vi "loadM300MachineStatusYY.vi"(10 "name or relative path":string="M420_LSTR機台狀況(早)_12月.xls", 11 "template (empty)":path=path "c:/m300") -> ()   [LabVIEW 2012]
uses:
  <vilib>/addons/database/Auxilliary.llb/DB Tools Cursor Type.ctl
  <vilib>/Utility/NIReport.llb/NI_report.lvclass
  <vilib>/addons/database/Connection.llb/DB Tools Open Connec (Path).vi
  <vilib>/addons/database/Connection.llb/Conn Execute.vi
  <vilib>/addons/database/Recordset.llb/Rec Destroy - Connection.vi
  <vilib>/addons/_office/excel.llb/Excel Get Data (str).vi
  <vilib>/addons/database/NI_Database_API.lvlib
  <vilib>/addons/_office/NI_ReportGenerationToolkit.lvlib
  <vilib>/Utility/NIReport.llb/Excel/NI_Excel.lvclass
panel:
  out "output cluster":T1
  out "error out 5":errorcluster
  out "error out":errorcluster
  out "after substring":string
  in  "array 2":string[][](array[string])
  in  "Cluster 2":T1
  out "error out 4":errorcluster
  out "error out 3":errorcluster
  in  "start (0, 0)":cluster{"start row":i32, "start column":i32}
  out "x+y":i32
  out "data":string
  in  "start (0, 0) 2":cluster{"start row":i32, "start column":i32}
  out "data 2":string
  in  "start (0, 0) 3":cluster{"start row":i32, "start column":i32}
  out "data 3":string
  out "Numeric":i32
  out "array":string[](array[string])
  out "x+y 2":i32
  out "x > y?":bool
  out "s? t:f":string
  out "concatenated string":string
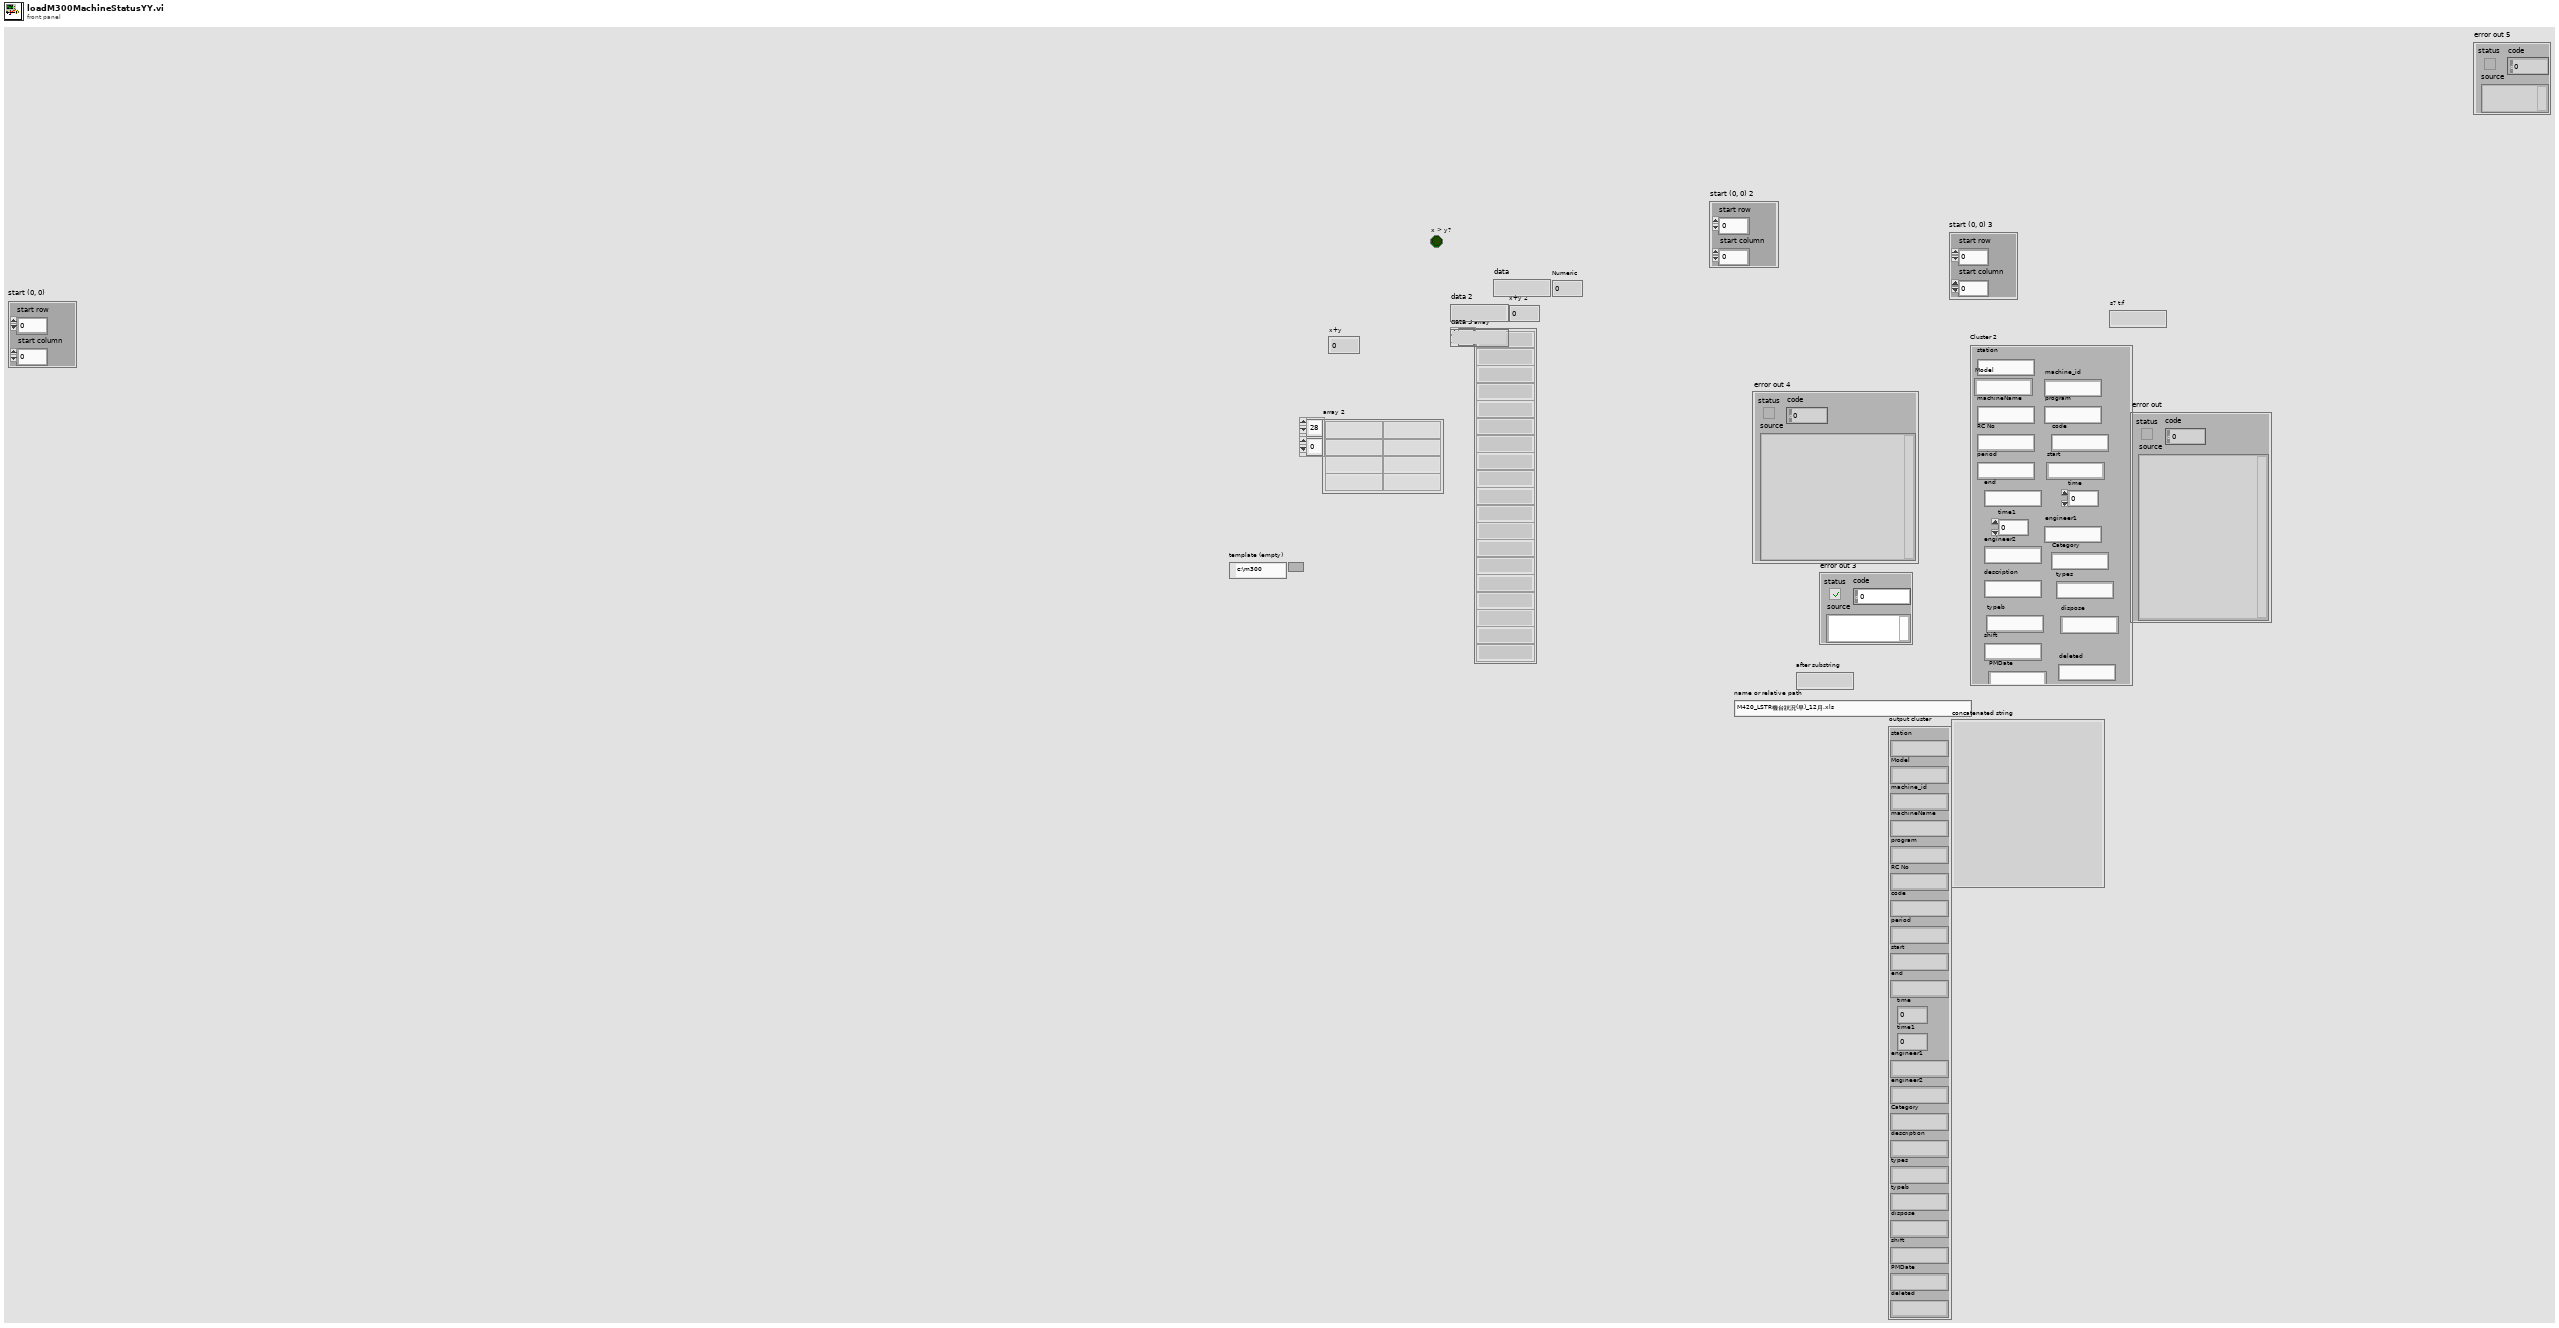
[diagram p1: front panel]
types:
  T1 = cluster{"station":string, "Model":string, "machine_id":string, "machineName":string, "program":string, "RC No":string, "code":string, "period":string, "start":string, "end":string, "time":dbl, "time1":dbl, "engineer1":string, "engineer2":string, "Category":string, "description":string, "types":string, "typeb":string, "dispose":string, "shift":string, "PMDate":string, "deleted":string}
  T2 = enum16{"Standard Report", "HTML", "Word", "Excel"}
  T3 = typedef "NI_Database_API.lvlib/Conn ObjectReference.ctl" = refnum<k1>
  T4 = typedef "NI_Database_API.lvlib/DB Tools Cursor Type.ctl" = enum16{"forward-only", "keyset", "dynamic", "static"}
  T5 = typedef "NI_Database_API.lvlib/Rec ObjectReference.ctl" = refnum<k1>
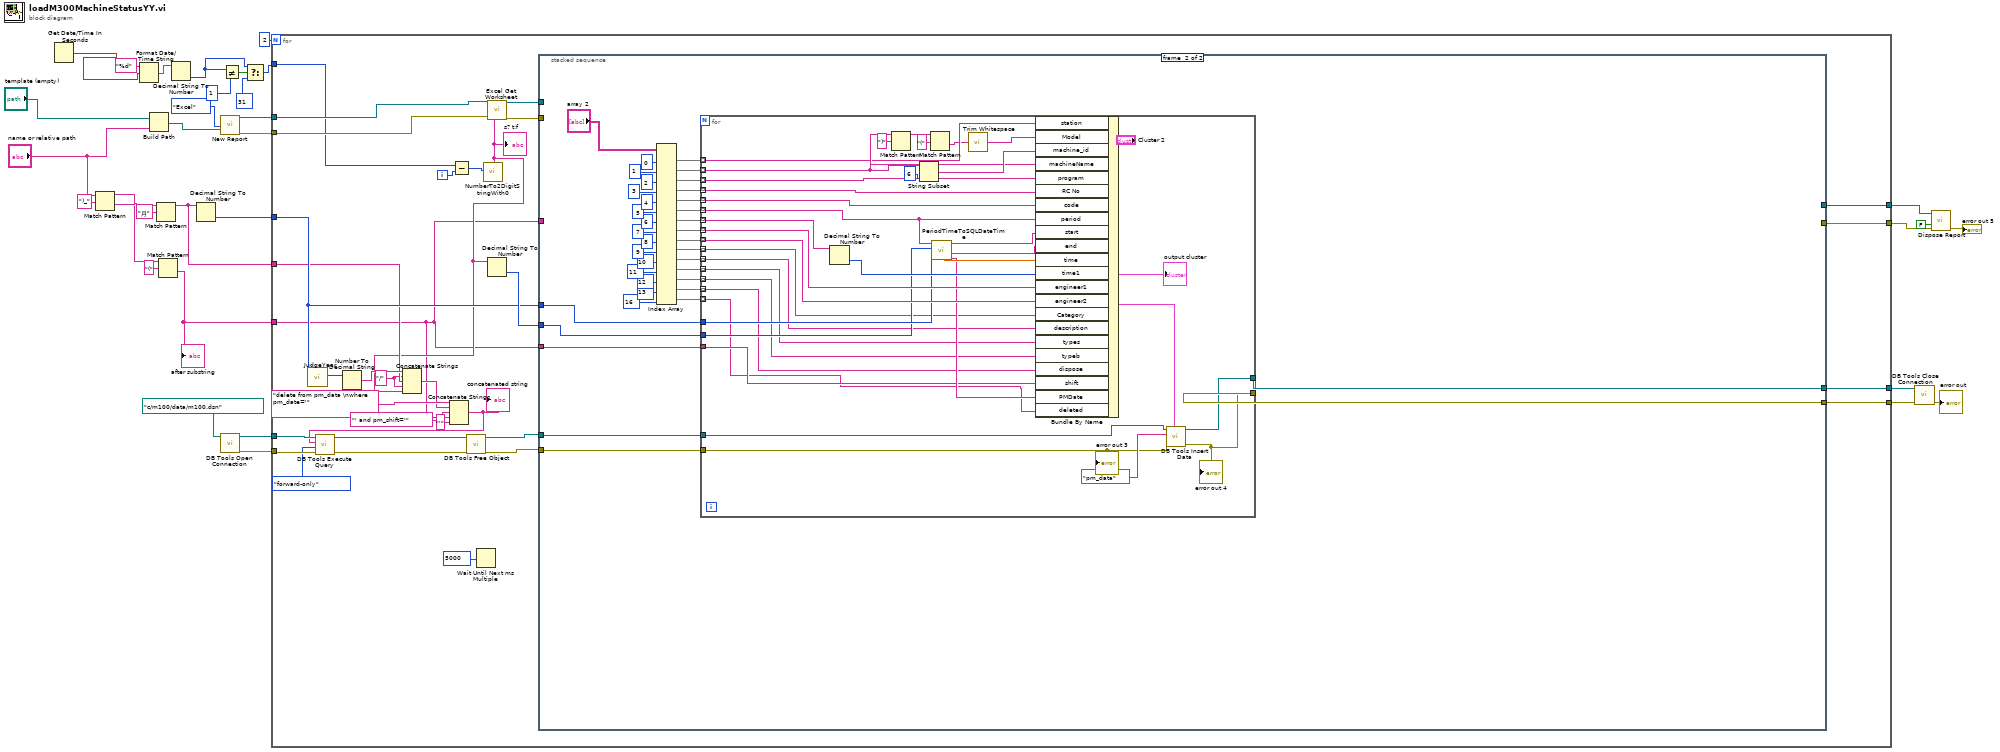
[diagram p0: block diagram]
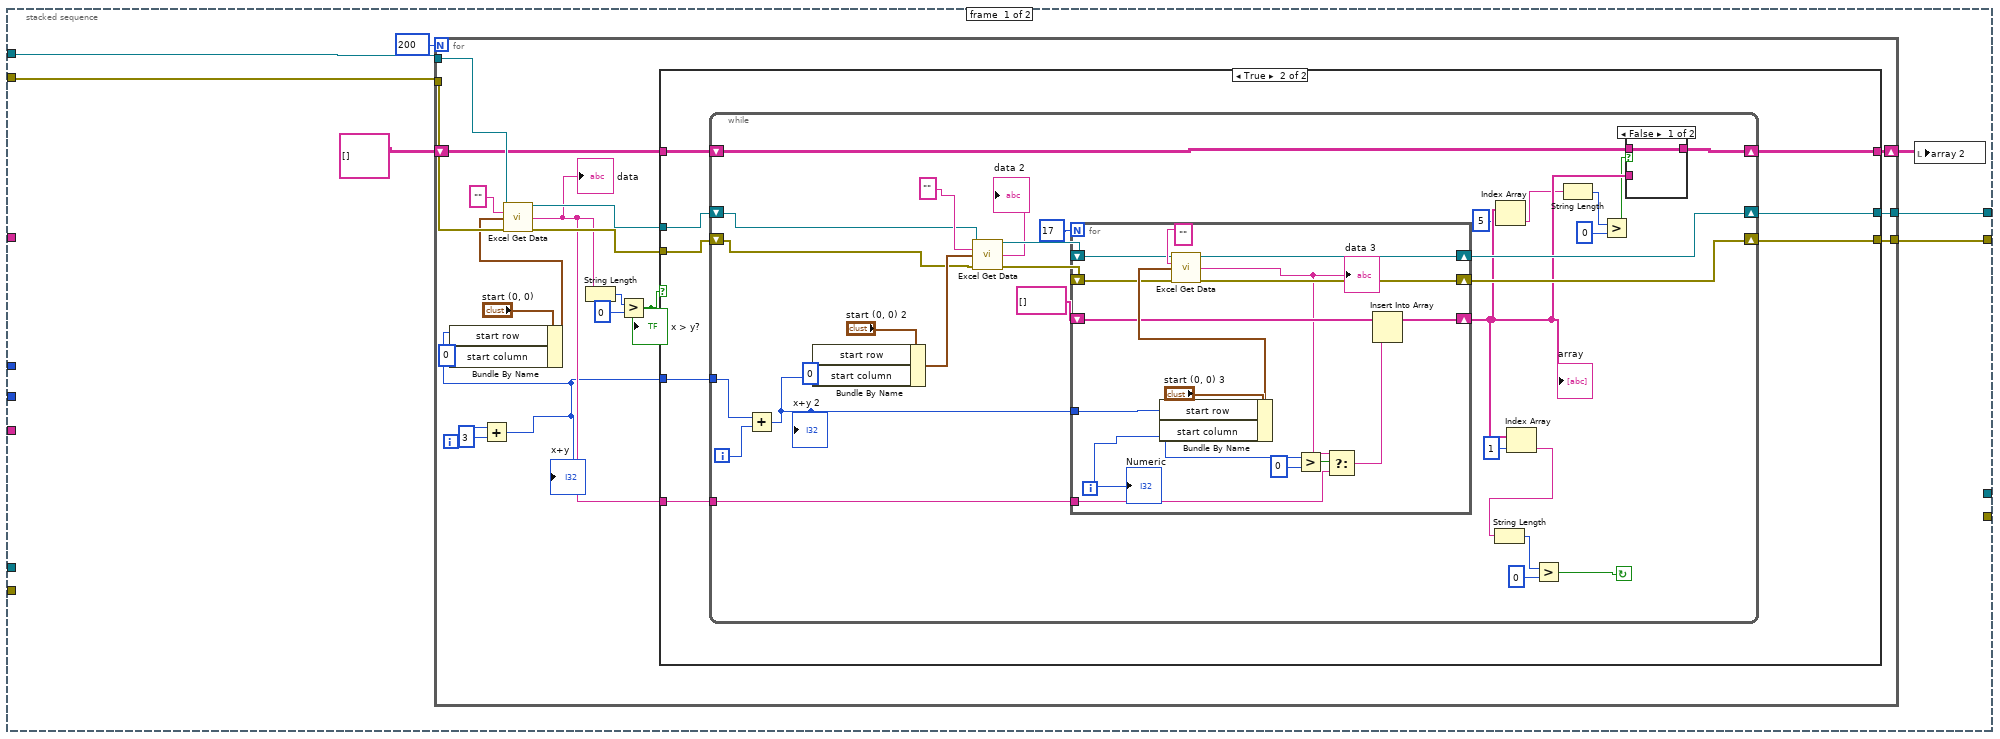
[diagram p2: hidden frame]
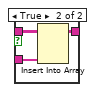
[diagram p4: hidden frame]
diagram:
  n1 = Get Date/Time In Seconds() -> (seconds since 1Jan1904=w22:timestamp)
  n2 = Match Pattern(string="name or relative path", regular expression=")_") -> (before substring=w26:string, after substring=w33:string)  [unwired: 1 in, 2 out]
  n3 = Format Date/Time String(time format string (%c)="%d", seconds (now)=w22) -> (date/time string=w23:string)  [unwired: 1 in]
  n4 = Build Path(base path="template (empty)", name or relative path="name or relative path") -> (appended path=w15:path)
  n5 = Match Pattern(string=w33, regular expression="月") -> (before substring=w10:string)  [unwired: 1 in, 3 out]
  n6 = Match Pattern(string=w26, regular expression="(") -> (after substring=w25:string)  [unwired: 1 in, 3 out]
  "after substring" <- w25
  n7 = Decimal String To Number(string=w23) -> (number=w18:i32)  [unwired: 2 in, 1 out]
  n8 = Decimal String To Number(string=w10) -> (number=w28:i32)  [unwired: 2 in, 1 out]
  n9 = call <vilib>:"New Report.vi"("report type"=T2."Excel" ("Report Type"), "template (empty)"=w15) -> ("report out"=w14:refnum<class "NI_report.lvclass">, "error out"=w13:errorcluster)  [unwired: 12 in]
  n10 = call-poly <vilib>:"DB Tools Open Connection.vi"("connection information"=path "c:/m100/data/m100.dsn") -> ("error out"=w11:errorcluster, "connection reference"=w12:T3)  [unwired: 7 in]
  n11 = Not Equal?(x=w18, y=1) -> (x != y?=w20:bool)
  n12 = Select(t=w18, s=w20, f=31) -> (s? t:f=w1:i32)
  n13 = for {
    N: 2 -> [_]
    tunnel: w28 -> [w59]
    tunnel: w25 -> [w39]
    tunnel: w14 -> [w61]
    tunnel: w13 -> [w60]
    tunnel: w12 -> [w41]
    tunnel: w11 -> [w43]
    tunnel: w10 -> [w56]
    tunnel: [w51] -> w8
    tunnel: [w50] -> w7
    tunnel: [w37] -> w4
    tunnel: [w36] -> w3
    tunnel: w1 -> [w35]
    i -> [w63]
    w55 = "/" ("string")
    n14 = call "JudgeYear.vi"("DataMonth"=w59) -> ("DataYear"=w58:i32)  [unwired: 10 in]
    n15 = Number To Decimal String(number=w58) -> (decimal integer string=w57:string)  [unwired: 1 in]
    n16 = Subtract(x=w35, y=w63) -> (x-y=w48:i32)
    n17 = Wait Until Next ms Multiple(millisecond multiple=u32 5000) -> ()  [unwired: 1 out]
    n18 = call "NumberTo2DigitStringWith0.vi"("number"=w48) -> ("s? t:f"=w49:string)  [unwired: 10 in]
    "s? t:f" <- w49
    n19 = Concatenate Strings(w57, w55, w56, w55, w49) -> (w53:string)
    n20 = Concatenate Strings("delete from pm_data \nwhere pm_date='" ("string"), w53, "' and pm_shift='" ("string"), w39, "'" ("string")) -> (w40:string)
    "concatenated string" <- w40
    n21 = call-poly <vilib>:"DB Tools Execute Query.vi"("error in (no error)"=w43, "cursor type"=DB_Tools_Cursor_Type."forward-only", "SQL query"=w40, "connection reference"=w41) -> ("error out"=w44:errorcluster, "recordset reference"=w45:T5)  [unwired: 4 in]
    n22 = call-poly <vilib>:"DB Tools Free Object.vi"("error in (no error)"=w44, "recordset reference"=w45) -> ("error out"=w46:errorcluster, "connection reference"=w47:T3)  [unwired: 8 in]
    n23 = call <vilib>:"Excel Get Worksheet.vi"("report in"=w61, "error in (no error)"=w60, "name (\"\")"=w49) -> ("report out"=w65:refnum<class "NI_report.lvclass">, "error out"=w64:errorcluster)  [unwired: 11 in]
    n24 = Decimal String To Number(string=w49) -> (number=w62:i32)  [unwired: 2 in, 1 out]
    n25 = stacked-sequence {
      tunnel: w65 -> [w69 _]
      tunnel: w64 -> [w68 _]
      tunnel: w59 -> [_ w176]
      tunnel: w62 -> [_ w175]
      tunnel: w39 -> [_ w174]
      tunnel: w39 -> [_ _]
      tunnel: w47 -> [_ w173]
      tunnel: w46 -> [_ w172]
      tunnel: [_ w171] -> w51
      tunnel: [_ w170] -> w50
      tunnel: [w67 _] -> w37
      tunnel: [w66 _] -> w36
      frame #0 {
        n26 = for {
          N: 200 -> [_]
          tunnel: w69 -> [w91]
          tunnel: w68 -> [w90]
          shift-right: [w78] -> w71
          shift-left: string[][] [] ("array") -> [w77]
          tunnel: [w74] -> w67
          tunnel: [w73] -> w66
          i -> [w86]
          n27 = Add(x=w86, y=3) -> (x+y=w75:i32)
          "x+y" <- w75
          n28 = Bundle By Name(cluster="start (0, 0)", "start row"=w75, "start column"=0) -> (w87:cluster{"start row":i32, "start column":i32})
          n29 = call-poly <vilib>:"Excel Get Data.vi"("report in"=w91, "data type"="", "start (0, 0)"=w87, "error in (no error)"=w90) -> ("report out"=w83:refnum<class "NI_report.lvclass">, "data"=w76:string, "error out"=w82:errorcluster)  [unwired: 9 in]
          "data" <- w76
          n30 = String Length(string=w76) -> (length=w81:i32)
          n31 = Greater?(x=w81, y=0) -> (0:w79:bool)
          "x > y?" <- w79
          n32 = case shown="True" w79 {
            tunnel: w75 -> [_ w102]
            tunnel: w83 -> [w93 w101]
            tunnel: w82 -> [w92 w100]
            tunnel: [w94 w99] -> w78
            tunnel: w77 -> [w94 w98]
            tunnel: w76 -> [_ w97]
            tunnel: [w93 w96] -> w74
            tunnel: [w92 w95] -> w73
            frame False {
            }
            frame True {
              n33 = while {
                tunnel: w102 -> [w131]
                shift-right: [w121] -> w99
                shift-left: w98 -> [w120]
                shift-right: [w119] -> w96
                shift-left: w101 -> [w117]
                shift-right: [w118] -> w95
                shift-left: w100 -> [w116]
                tunnel: w97 -> [w103]
                i -> [w130]
                stop <- w111 continue-if-true
                n34 = Add(x=w131, y=w130) -> (x+y=w124:i32)
                "x+y 2" <- w124
                n35 = Bundle By Name(cluster="start (0, 0) 2", "start row"=w124, "start column"=0) -> (w129:cluster{"start row":i32, "start column":i32})
                n36 = call-poly <vilib>:"Excel Get Data.vi"("report in"=w117, "data type"="", "start (0, 0)"=w129, "error in (no error)"=w116) -> ("report out"=w125:refnum<class "NI_report.lvclass">, "data"=→"data 2":string, "error out"=w126:errorcluster)  [unwired: 9 in]
                n37 = for {
                  N: 17 -> [_]
                  shift-right: [w149] -> w119
                  shift-left: w125 -> [w147]
                  shift-right: [w148] -> w118
                  shift-left: w126 -> [w146]
                  tunnel: w124 -> [w143]
                  shift-right: [w145] -> w110
                  shift-left: string[] [] ("array") -> [w144]
                  tunnel: w103 -> [w137]
                  i -> [w142]
                  n38 = Bundle By Name(cluster="start (0, 0) 3", "start row"=w143, "start column"=w142) -> (w151:cluster{"start row":i32, "start column":i32})
                  n39 = call-poly <vilib>:"Excel Get Data.vi"("report in"=w147, "data type"="", "start (0, 0)"=w151, "error in (no error)"=w146) -> ("report out"=w149:refnum<class "NI_report.lvclass">, "data"=w139:string, "error out"=w148:errorcluster)  [unwired: 9 in]
                  "data 3" <- w139
                  n40 = Greater?(x=w142, y=0) -> (0:w140:bool)
                  n41 = Select(t=w139, s=w140, f=w137) -> (s? t:f=w138:string)
                  n42 = Insert Into Array(array=w144, new element=w138) -> (w145:string[])  [unwired: 1 in]
                  "Numeric" <- w142
                }
                "array" <- w110
                n43 = Index Array(array=w110, index=5) -> (element=w106:string)
                n44 = Index Array(array=w110, index=1) -> (element=w112:string)
                n45 = String Length(string=w112) -> (length=w115:i32)
                n46 = Greater?(x=w115, y=0) -> (0:w111:bool)
                n47 = String Length(string=w106) -> (length=w108:i32)
                n48 = Greater?(x=w108, y=0) -> (0:w105:bool)
                n49 = case shown="False" w105 {
                  tunnel: [w133 w136] -> w121
                  tunnel: w120 -> [w133 w135]
                  tunnel: w110 -> [_ w134]
                  frame False {
                  }
                  frame True {
                    n50 = Insert Into Array(array=w135, new element=w134) -> (w136:string[][])  [unwired: 2 in]
                  }
                }
              }
            }
          }
        }
        n51 = local write "array 2"(w71) -> ()
      }
      frame #1 {
        n52 = Index Array(array="array 2", index (col) #1=0 ("disabled index (col)"), index (col) #2=1 ("index (col)"), index (col) #3=2 ("index (col)"), index (col) #4=3 ("index (col)"), index (col) #5=4 ("index (col)"), index (col) #6=5 ("index (col)"), index (col) #7=6 ("index (col)"), index (col) #8=7 ("index (col)"), index (col) #9=8 ("index (col)"), index (col) #10=9 ("index (col)"), index (col) #11=10 ("index (col)"), index (col) #12=11 ("index (col)"), index (col) #13=12 ("index (col)"), index (col) #14=13 ("index (col)"), index (col) #15=16 ("index (col)")) -> (element #1=w189:string[], element #2=w188:string[], element #3=w187:string[], element #4=w186:string[], element #5=w185:string[], element #6=w184:string[], element #7=w183:string[], element #8=w182:string[], element #9=w181:string[], element #10=w180:string[], element #11=w179:string[], element #12=w178:string[], element #13=w177:string[], element #14=w169:string[], element #15=w153:string[])  [unwired: 15 in]
        n53 = for {
          tunnel: w189 -> [w204] mode=indexing
          tunnel: w188 -> [w205] mode=indexing
          tunnel: w187 -> [w225] mode=indexing
          tunnel: w186 -> [w224] mode=indexing
          tunnel: w185 -> [w223] mode=indexing
          tunnel: w184 -> [w209] mode=indexing
          tunnel: w183 -> [w221] mode=indexing
          tunnel: w182 -> [w220] mode=indexing
          tunnel: w181 -> [w219] mode=indexing
          tunnel: w180 -> [w192] mode=indexing
          tunnel: w179 -> [w193] mode=indexing
          tunnel: w178 -> [w194] mode=indexing
          tunnel: w177 -> [w195] mode=indexing
          tunnel: [w214] -> w171
          tunnel: [w213] -> w170
          tunnel: w176 -> [w211]
          tunnel: w175 -> [w210]
          tunnel: w174 -> [w197]
          tunnel: w173 -> [w200]
          tunnel: w172 -> [w199]
          tunnel: w169 -> [w196] mode=indexing
          tunnel: w153 -> [w191] mode=indexing
          n54 = Decimal String To Number(string=w221) -> (number=w218:i32)  [unwired: 2 in, 1 out]
          n55 = Match Pattern(string=w205, regular expression=")") -> (before substring=w206:string)  [unwired: 1 in, 3 out]
          n56 = String Subset(string=w205, length (rest)=6 ("length (rest)")) -> (substring=w226:string)  [unwired: 1 in]
          n57 = Match Pattern(string=w206, regular expression="(") -> (after substring=w202:string)  [unwired: 1 in, 3 out]
          n58 = call "PeriodTimeToSQLDateTime.vi"("day"=w210, "Month"=w211, "string"=w209) -> ("StingDate"=w198:string, "SQLDatetime2"=w216:string, "SQLDateTime1"=w217:string, "Period(M)"=w215:dbl)  [unwired: 5 in]
          n59 = call <vilib>:"Trim Whitespace.vi"("string"=w202) -> ("trimmed string"=w203:string)  [unwired: 1 in]
          n60 = Bundle By Name(cluster="Cluster 2", "station"=w204, "Model"=w203, "machine_id"=w226, "machineName"=w205, "program"=w225, "RC No"=w224, "code"=w223, "period"=w209, "start"=w217, "end"=w216, "time"=w215, "time1"=w218, "engineer1"=w220, "engineer2"=w219, "Category"=w192, "description"=w193, "types"=w194, "typeb"=w195, "dispose"=w196, "shift"=w197, "PMDate"=w198, "deleted"=w191) -> (w212:T1)
          "output cluster" <- w212
          n61 = call <vilib>:"DB Tools Insert Data.vi"("data"=w212, "error in (no error)"=w199, "table"="pm_data", "connection reference"=w200) -> ("error out"=w213:errorcluster, "connection reference out"=w214:T3)  [unwired: 6 in]
          "error out 4" <- w213
          "error out 3" <- w199
        }
      }
    }
  }
  n62 = call <vilib>:"DB Tools Close Connection.vi"("error in (no error)"=w7, "connection reference"=w8) -> ("error out"=→"error out":errorcluster)  [unwired: 5 in]
  n63 = call-dynamic "Dispose Report.vi"("report in"=w4, "save changes? (F)"=FALSE, "error in (no error)"=w3) -> ("error out"=→"error out 5":errorcluster)  [unwired: 12 in]
